vi "labview_toggle_with_watchdog.vi"() -> ()   [LabVIEW 2026]
panel:
  out "Serial Monitor":string
  out "LED Status":bool
  in  "LED Toggle":bool
  in  "Cancel Program":bool
  out "ESP32 Status":bool
  in  "Serial Port":refnum<visa-resource-name>
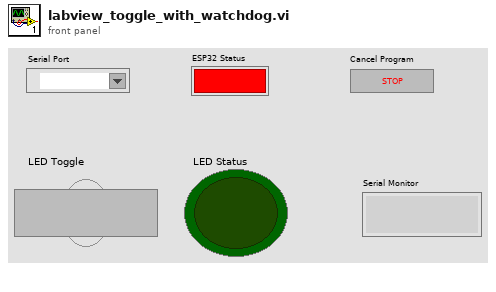
[diagram p1: front panel]
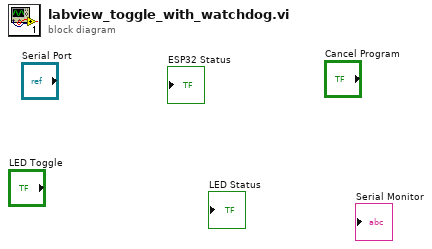
[diagram p0: block diagram]
diagram:
